vi "SetParam.vi"(8 "error in (no error)":errorcluster caption="entrée d'erreur (pas d'erreur)", 10 "LeavePGroupsOut":cluster{"n_groups":i32}={"n_groups"=2}, 11 "LeavePGroupsOut.lvclass":refnum<class "LeavePGroupsOut.lvclass">) -> (0 "error out":errorcluster caption="sortie d'erreur", 3 "LeavePGroupsOut.lvclass":refnum<class "LeavePGroupsOut.lvclass">)   [LabVIEW 2020, in "LeavePGroupsOut.lvclass"]
doc: "Set Parameters"
uses:
  LeavePGroupsOut.lvclass
  LeavePGroupsOut.lvclass/LeavePGroupsOut.ctl
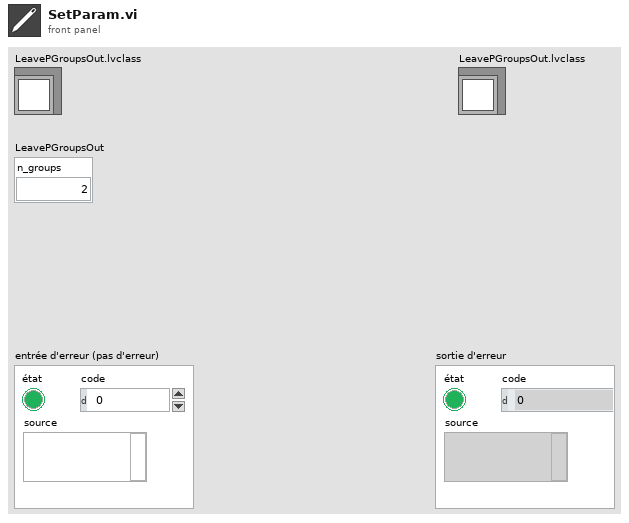
[diagram p1: front panel]
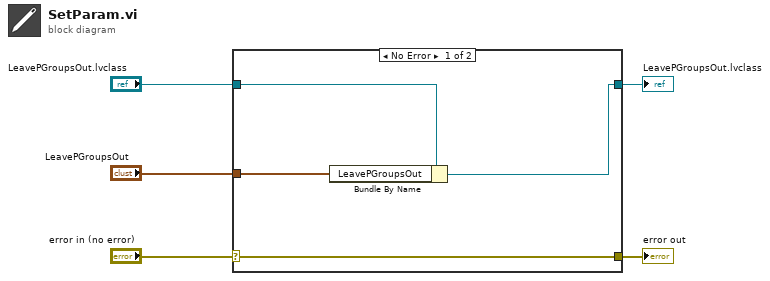
[diagram p0: block diagram]
diagram:
  n1 = case shown="No Error" "error in (no error)" {
    selector: "error in (no error)" -> [w9 w10]
    tunnel: [w9 w10] -> w4
    tunnel: [w7 w11] -> w2
    tunnel: "LeavePGroupsOut.lvclass" -> [w8 w11]
    tunnel: "LeavePGroupsOut" -> [w6 _]
    frame No Error {
      n2 = Bundle By Name(cluster=w8, "LeavePGroupsOut"=w6) -> (w7:refnum<class "LeavePGroupsOut.lvclass">)
    }
    frame Error {
    }
  }
  "error out" <- w4
  "LeavePGroupsOut.lvclass" <- w2
